vi "DriveToTarget.vi"(8 "error in":errorcluster) -> (0 "error out":errorcluster)   [LabVIEW 2020]
doc: "Drives robot to peg or gear and stops"
uses:
  Framework/Robot Global Data.vi
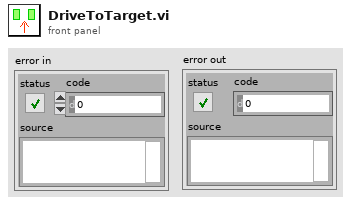
[diagram p1: front panel]
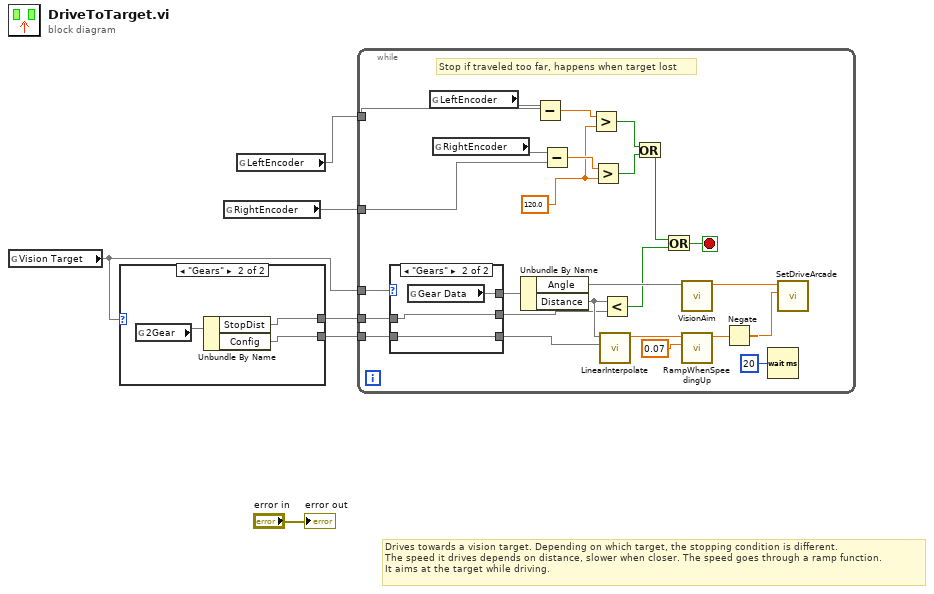
[diagram p0: block diagram]
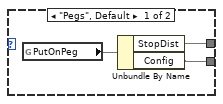
[diagram p2: hidden frame]
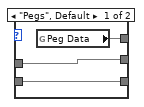
[diagram p3: hidden frame]
diagram:
  # "Drives towards a vision target. Depending on which target, the stopping condition is different.\nThe speed it drives depends on distance, slower when closer. The speed goes through a ramp function.\nIt aims at the target while driving."
  n1 = global read "Robot Global Data.vi" "Vision Target"() -> (w5)
  n2 = case shown="\"Gears\"" w5 {
    tunnel: [w8 w11] -> w4
    tunnel: [w7 w10] -> w3
    frame "Pegs", Default {
      n3 = global read "Robot Global Data.vi" "PutOnPeg"() -> (w9)
      n4 = Unbundle By Name(w9) -> ("StopDist"=w8, "Config"=w7)
    }
    frame "Gears" {
      n5 = global read "Robot Global Data.vi" "2Gear"() -> (w12)
      n6 = Unbundle By Name(w12) -> ("StopDist"=w11, "Config"=w10)
    }
  }
  n7 = global read "Robot Global Data.vi" "RightEncoder"() -> (w1)
  n8 = global read "Robot Global Data.vi" "LeftEncoder"() -> (w2)
  n9 = while {
    tunnel: w5 -> [w38]
    tunnel: w4 -> [w26]
    tunnel: w3 -> [w25]
    tunnel: w2 -> [w22]
    tunnel: w1 -> [w21]
    stop <- w13 stop-if-true
    w18 = 120.0 ("Max Rate")
    # "Stop if traveled too far, happens when target lost"
    n10 = case shown="\"Gears\"" w38 {
      tunnel: [w41 w44] -> w37
      tunnel: [w40 w43] -> w33
      tunnel: [w39 w42] -> w28
      tunnel: w26 -> [w40 w43]
      tunnel: w25 -> [w39 w42]
      frame "Pegs", Default {
        n11 = global read "Robot Global Data.vi" "Peg Data"() -> (w41)
      }
      frame "Gears" {
        n12 = global read "Robot Global Data.vi" "Gear Data"() -> (w44)
      }
    }
    n13 = global read "Robot Global Data.vi" "LeftEncoder"() -> (w24)
    n14 = global read "Robot Global Data.vi" "RightEncoder"() -> (w23)
    n15 = Unbundle By Name(w37) -> ("Angle"=w36, "Distance"=w34)
    n16 = Subtract(x=w24, y=w22) -> (x-y=w20:dbl)
    n17 = Subtract(x=w23, y=w21) -> (x-y=w19:dbl)
    n18 = Greater?(x=w20, y=w18) -> (0:w16:bool)
    n19 = Greater?(x=w19, y=w18) -> (0:w17:bool)
    n20 = call "LinearInterpolate.vi"("Points"=w28, "Value"=w34) -> ("Output"=w32:dbl)  [unwired: 9 in]
    n21 = Less?(x=w34, y=w33) -> (x < y?=w14:bool)
    n22 = Or(x=w16, y=w17) -> (x .or. y?=w15:bool)
    n23 = Or(x=w15, y=w14) -> (x .or. y?=w13:bool)
    n24 = call "VisionAim.vi"("Angle"=w36) -> ("Turn"=w35:dbl)  [unwired: 9 in, 1 out]
    n25 = call "RampWhenSpeedingUp.vi"("Ramp"=0.07 ("Max Rate"), "Input"=w32) -> ("Output"=w30:dbl)  [unwired: 9 in]
    n26 = Negate(x=w30) -> (-x=w29:dbl)
    n27 = Wait (ms)(milliseconds to wait=u32 20) -> ()  [unwired: 1 out]
    n28 = call "SetDriveArcade.vi"("Forward"=w29, "Turn"=w35) -> ()  [unwired: 9 in, 1 out]
  }
  "error out" <- "error in"
